vi "Destroy MIDI In Event.vi"(8 "error in (no error)":errorcluster, 11 "MIDI":refnum<user-event>) -> (0 "error out":errorcluster)   [LabVIEW 2020, in "MIDIllan.lvlib" / "midi in.lvclass"]
uses:
  midi in.lvclass
  MIDIin.ctl
  Message Type.ctl
  midi in.lvclass/midi in.ctl
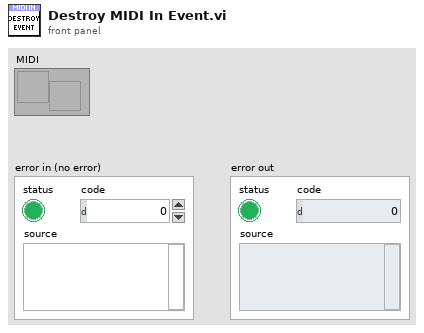
[diagram p1: front panel]
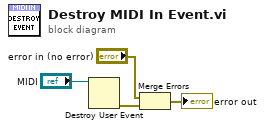
[diagram p0: block diagram]
diagram:
  n1 = Destroy User Event(user event="MIDI") -> (error out=w4:errorcluster)  [unwired: 1 in]
  n2 = Merge Errors("error in (no error)", w4) -> (→"error out":errorcluster)
